vi "test python.vi"() -> ()   [LabVIEW 2019]
panel:
  in  "error in (no error)":errorcluster
  out "error out":errorcluster
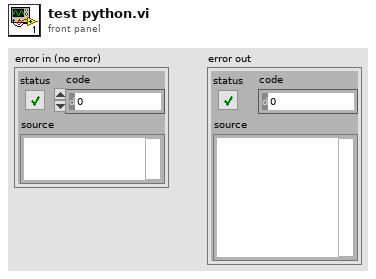
[diagram p1: front panel]
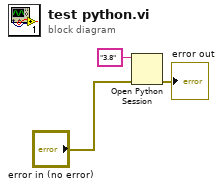
[diagram p0: block diagram]
diagram:
  n1 = Open Python Session(python version="3.8" ("Python version"), 3:"error in (no error)") -> (error out=→"error out":errorcluster)  [unwired: 1 in, 1 out]
